vi "Close Panel.vi"(8 "error in (no error)":errorcluster, 10 "Panel":refnum<class "Panel.lvclass">, 11 "Manager in":refnum<class "Manager.lvclass">) -> (0 "error out":errorcluster, 3 "Manager out":refnum<class "Manager.lvclass">)   [LabVIEW 2020, in "OOPanel.lvlib" / "Manager.lvclass"]
uses:
  Manager.lvclass
  Panel/Panel.lvclass
  Panel/Close Reason.ctl
  Manager.lvclass/Manager.ctl
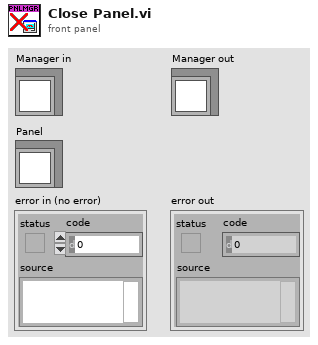
[diagram p1: front panel]
types:
  T1 = typedef "OOPanel.lvlib/Panel.lvclass/Close Reason.ctl" = enum16{"Shutdown", "Close"}
  T2 = typedef "OOPanel.lvlib/Panel.lvclass/Visibility State.ctl" = enum16{"Idle", "Closed", "Hidden", "Visible", "Subpanel"}
  T3 = typedef "OOPanel.lvlib/Manager.lvclass/Ref Data.ctl" = cluster{"SubPanel Map":T4, "Panels":refnum<class "Panel.lvclass">[]}
  T4 = typedef "OOPanel.lvlib/Manager.lvclass/SubPanel Map.ctl" = cluster{"SubPanels":refnum<vi>[], "Panels":refnum<class "Panel.lvclass">[]}
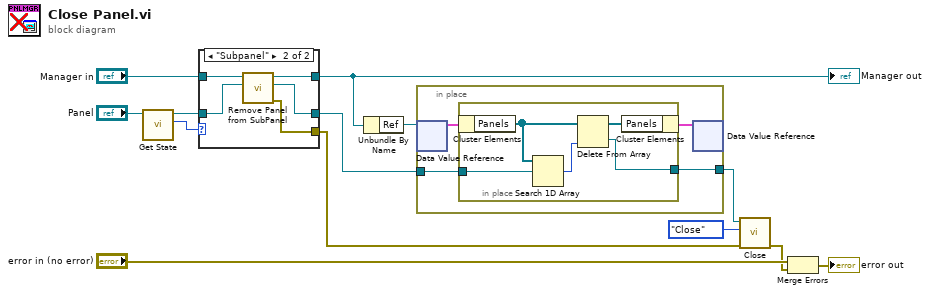
[diagram p0: block diagram]
diagram:
  n1 = call "Get State.vi"("Panel in"="Panel") -> ("State"=w11:T2, "Panel out"=w10:refnum<class "Panel.lvclass">)  [unwired: 8 in, 1 out]
  n2 = case shown="\"Subpanel\"" w11 {
    tunnel: w10 -> [w15 w19]
    tunnel: "Manager in" -> [w14 w20]
    tunnel: [w14 w18] -> w7
    tunnel: [w15 w17] -> w6
    tunnel: [_ w16] -> w5
    frame Default {
    }
    frame "Subpanel" {
      n3 = call "Remove Panel from SubPanel.vi"("Panel In"=w19, "Manager in"=w20) -> ("error out"=w16:errorcluster, "Panel"=w17:refnum<class "Panel.lvclass">, "Manager out"=w18:refnum<class "Manager.lvclass">)  [unwired: 7 in]
    }
  }
  "Manager out" <- w7
  n4 = Unbundle By Name(w7) -> ("Ref"=w8:refnum<data-value>)
  n5 = in-place {
    in-place-border: w6 -> [w22]
    in-place-border: [w21] -> w4
    n6 = in-place-dvr #1(w8) -> (w24:T3)  [unwired: 1 out]
    n7 = in-place {
      in-place-border: w22 -> [w29]
      in-place-border: [w25] -> w21
      n8 = in-place-cluster #2(w24) -> ("Panels"=w28:refnum<class "Panel.lvclass">[])
      n9 = Search 1D Array(1D array=w28, element=w29) -> (index of element=w27:i32)  [unwired: 1 in]
      n10 = Delete From Array(array=w28, index=w27) -> (deleted portion=w25:refnum<class "Panel.lvclass">, array with subset deleted=w26:refnum<class "Panel.lvclass">[])  [unwired: 1 in]
      n11 = in-place-cluster #2("Panels"=w26) -> (w23:T3)
    }
    n12 = in-place-dvr #1(w23) -> ()  [unwired: 2 out]
  }
  n13 = call "Close.vi"("error in (no error)"=w5, "Reason"=Close_Reason."Close", "Panel in"=w4) -> ("error out"=w1:errorcluster)  [unwired: 7 in, 1 out]
  n14 = Merge Errors("error in (no error)", w1) -> (→"error out":errorcluster)
